vi "Day 8 Puzzle 1.vi"(11 "Path":path) -> ()   [LabVIEW 2021]
uses:
  <vilib>/Utility/file.llb/Read Delimited Spreadsheet (string).vi
panel:
  out "sum":i32
  out "Array":bool[][](array[boolean])
  out "Numeric":i32
  out "Array":bool[][](array[boolean])
  out "Number of rows":i32
  out "Number of columns":i32
  out "Grid array":i32[][](array[numeric])
  out "subarray":string[](array[string])
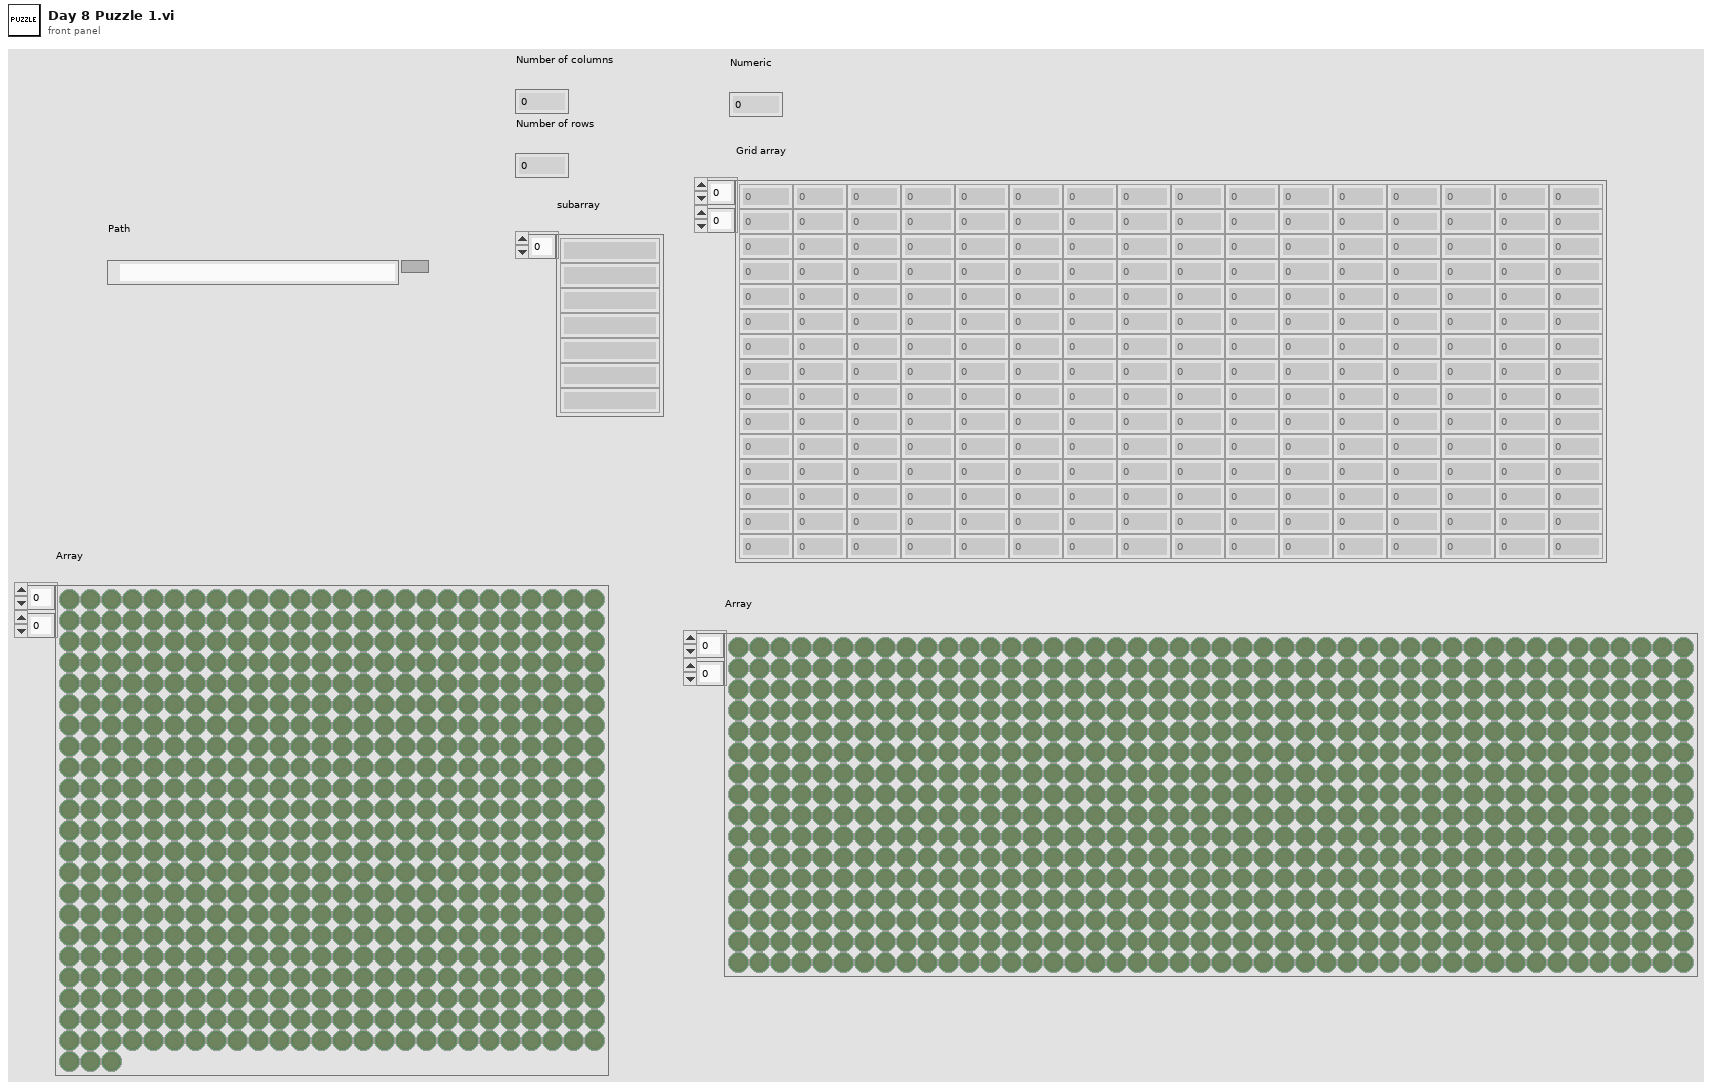
[diagram p1: front panel]
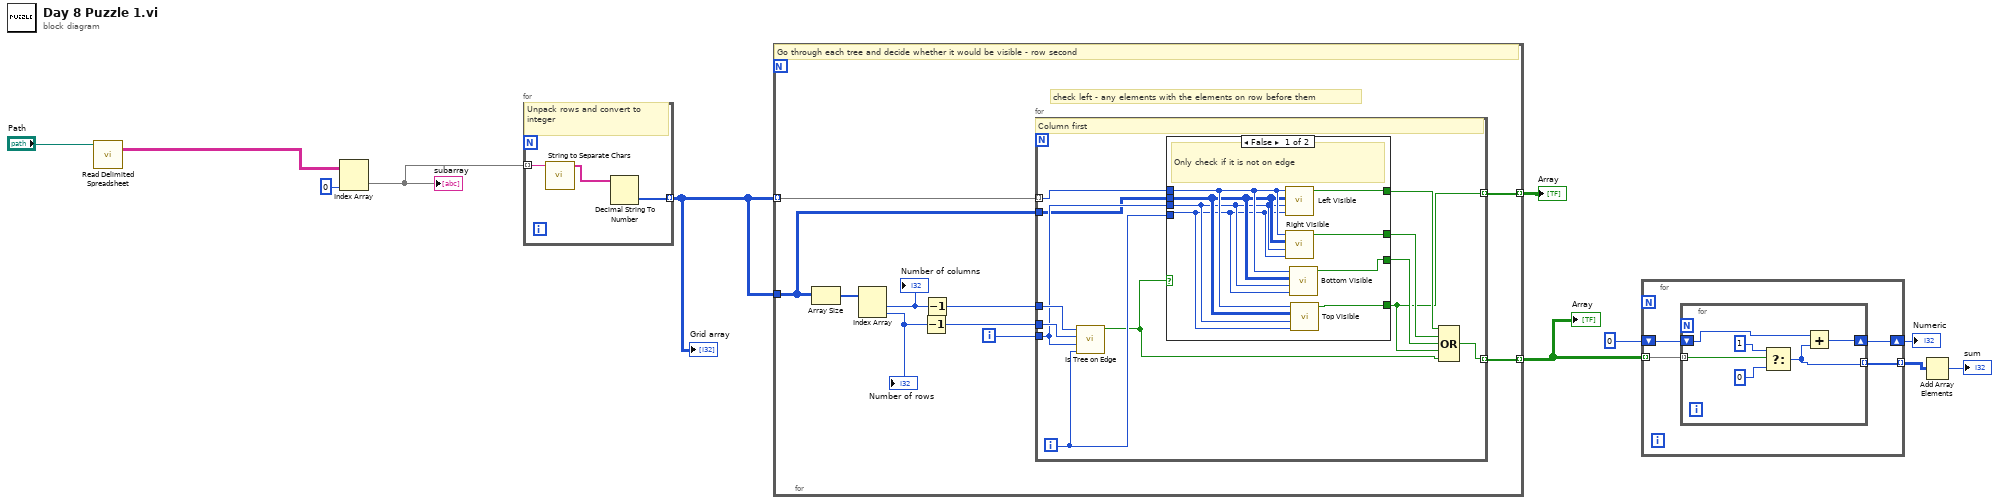
[diagram p0: block diagram]
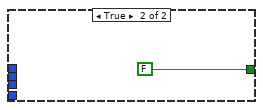
[diagram p2: hidden frame]
diagram:
  n1 = call-poly <vilib>:"Read Delimited Spreadsheet.vi"("file path (dialog if empty)"="Path") -> ("all rows"=w10:string[][])  [unwired: 9 in, 5 out]
  n2 = Index Array(array=w10, index (col)=0 ("disabled index (col)")) -> (element=w8:string[])  [unwired: 1 in]
  "subarray" <- w8
  n3 = for {
    tunnel: w8 -> [w14] mode=indexing
    tunnel: [w12] -> w7 mode=indexing
    # "Unpack rows and convert to integer"
    n4 = call "String to Separate Chars.vi"("String"=w14) -> ("Array"=w13:string[])  [unwired: 10 in]
    n5 = Decimal String To Number(string=w13) -> (number=w12:i32[])  [unwired: 2 in, 1 out]
  }
  "Grid array" <- w7
  n6 = for {
    tunnel: w7 -> [w23] mode=indexing
    tunnel: w7 -> [w16]
    tunnel: [w20] -> w3 mode=indexing
    tunnel: [w15] -> w4 mode=indexing
    i -> [w19]
    # "check left - any elements with the elements on row before them"
    # "Go through each tree and decide whether it would be visible - row second"
    n7 = Array Size(array=w16) -> (size(s)=w24:i32[])
    n8 = Index Array(array=w24) -> (element #1=w22:i32, element #2=w18:i32)  [unwired: 2 in]
    "Number of columns" <- w22
    "Number of rows" <- w18
    n9 = Decrement(x=w18) -> (x-1=w17:i32)
    n10 = Decrement(x=w22) -> (x-1=w21:i32)
    n11 = for {
      tunnel: w23 -> [w33] mode=indexing
      tunnel: w21 -> [w36]
      tunnel: [w31] -> w20 mode=indexing
      tunnel: w19 -> [w34]
      tunnel: w17 -> [w35]
      tunnel: w16 -> [w32]
      tunnel: [w25] -> w15 mode=indexing
      i -> [w30]
      # "Column first"
      n12 = call "Is Tree on Edge"("current row"=w30, "corrent column"=w34, "number of rows"=w35, "number of columns"=w36) -> ("Is on edge?"=w29:bool)  [unwired: 7 in]
      n13 = case shown="False" w29 {
        tunnel: w34 -> [w39 _]
        tunnel: w33 -> [w41 _]
        tunnel: w32 -> [w40 _]
        tunnel: [w44 FALSE ("Visible")] -> w27
        tunnel: w30 -> [w38 _]
        tunnel: [w43 _] -> w28
        tunnel: [w42 _] -> w26
        tunnel: [w37 _] -> w25
        frame False {
          # "Only check if it is not on edge"
          n14 = call "Left Visible.vi"("Current column"=w38, "Current row"=w39, "Full array"=w40, "Element"=w41) -> ("Visible"=w44:bool)  [unwired: 6 in, 1 out]
          n15 = call "Right Visible.vi"("Current column"=w38, "Current row"=w39, "Full array"=w40, "Element"=w41) -> ("Visible"=w43:bool)  [unwired: 6 in, 1 out]
          n16 = call "Bottom Visible.vi"("Current column"=w38, "Current row"=w39, "Full array"=w40, "Element"=w41) -> ("Visible"=w42:bool)  [unwired: 6 in, 1 out]
          n17 = call "Top Visible.vi"("Current column"=w38, "Current row"=w39, "Full array"=w40, "Element"=w41) -> ("Visible"=w37:bool)  [unwired: 6 in, 1 out]
        }
        frame True {
        }
      }
      n18 = Compound Arithmetic op=OR(w27, w28, w26, w25, w29) -> (w31:bool)
    }
  }
  "Array" <- w3
  "Array" <- w4
  n19 = for {
    tunnel: w3 -> [w49] mode=indexing
    shift-right: [w47] -> w5
    shift-left: 0 -> [w48]
    tunnel: [w46] -> w2 mode=indexing
    n20 = for {
      tunnel: w49 -> [w53] mode=indexing
      shift-right: [w51] -> w47
      shift-left: w48 -> [w52]
      tunnel: [w50] -> w46 mode=indexing
      n21 = Select(t=1, s=w53, f=0) -> (s? t:f=w50:i32)
      n22 = Add(x=w52, y=w50) -> (x+y=w51:i32)
    }
  }
  "Numeric" <- w5
  n23 = Add Array Elements(numeric array=w2) -> (sum=→"sum":i32)
